vi "VP.vi"(8 "error in (no error)":errorcluster caption="エラー入力（エラーなし）", 10 "文字待機 (200 ms)":u16=200, 11 "VISAリソース名":refnum<visa-resource-name>) -> (0 "error out":errorcluster caption="エラー出力", 2 "Motor count":i32, 3 "VISAリソース名（出力）":refnum<visa-resource-name>)   [LabVIEW 2017]
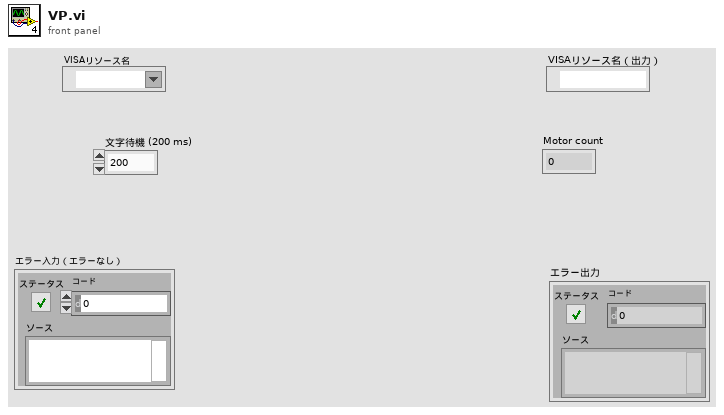
[diagram p1: front panel]
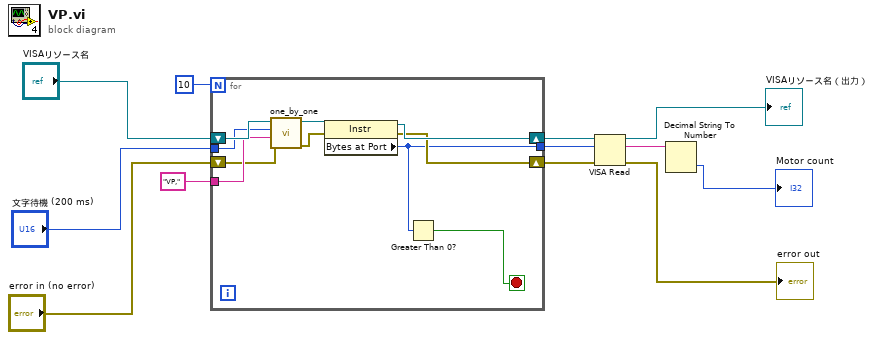
[diagram p0: block diagram]
diagram:
  n1 = for {
    N: 10 -> [_]
    tunnel: [w13] -> w12
    tunnel: "VP," -> [w17]
    tunnel: "文字待機 (200 ms)" -> [w16]
    shift-right: [w20] -> w11
    shift-left: "VISAリソース名" -> [w18]
    shift-right: [w19] -> w10
    shift-left: "error in (no error)" -> [w15]
    stop <- w14 stop-if-true
    n2 = call "one_by_one.vi"("error in (no error)"=w15, "入力文字"=w17, "待機 (200ms)"=w16, "VISAリソース名"=w18) -> ("error out"=w21:errorcluster, "VISAリソース名出力"=w22:refnum<visa-resource-name>)  [unwired: 6 in]
    n3 = property class="Instr"(reference=w22, error in=w21) -> (reference out=w20:refnum<visa-resource-name>, error out=w19:errorcluster, "Bytes at Port"=w13:u32)
    n4 = Greater Than 0?(x=w13) -> (x > 0?=w14:bool)
  }
  n5 = VISA Read(VISA resource name=w11, byte count=w12, error in (no error)=w10) -> (VISA resource name out=→"VISAリソース名（出力）":refnum<visa-resource-name>, read buffer=w9:string, error out=→"error out":errorcluster)  [unwired: 1 out]
  n6 = Decimal String To Number(string=w9) -> (number=→"Motor count":i32)  [unwired: 2 in, 1 out]
